vi "Top segment value_test3.vi"(10 "Top player segment position":string) -> (1 "Top player segment value":i32, 2 "Top player court segment display":bool[][](array[boolean]))   [LabVIEW 2014]
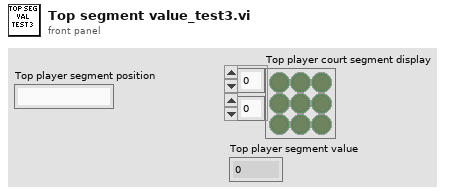
[diagram p1: front panel]
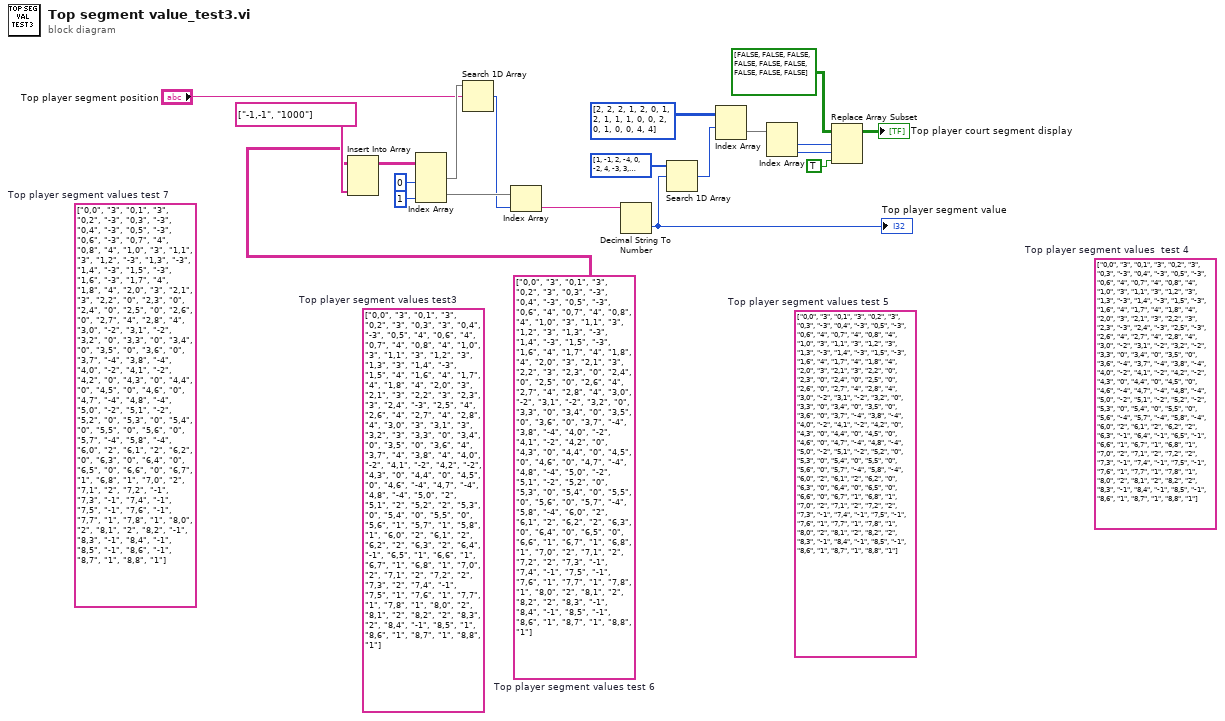
[diagram p0: block diagram]
diagram:
  (unwired) string[][] [["0,0", "3"], ["0,1", "3"], ["0,2", "-3"], ["0,3", "-3"], ["0,4", "-3"], ["0,5", "-3"], ["0,6", "-3"], ["0,7", "4"], ["0,8", "4"], ["1,0", "3"], ["1,1", "3"], ["1,2", "-3"], ["1,3", "-3"], ["1,4", "-3"], ["1,5", "-3"], ["1,6", "-3"], ["1,7", "4"], ["1,8", "4"], ["2,0", "3"], ["2,1", "3"], ["2,2", "0"], ["2,3", "0"], ["2,4", "0"], ["2,5", "0"], ["2,6", "0"], ["2,7", "4"], ["2,8", "4"], ["3,0", "-2"], ["3,1", "-2"], ["3,2", "0"], ["3,3", "0"], ["3,4", "0"], ["3,5", "0"], ["3,6", "0"], ["3,7", "-4"], ["3,8", "-4"], ["4,0", "-2"], ["4,1", "-2"], ["4,2", "0"], ["4,3", "0"], ["4,4", "0"], ["4,5", "0"], ["4,6", "0"], ["4,7", "-4"], ["4,8", "-4"], ["5,0", "-2"], ["5,1", "-2"], ["5,2", "0"], ["5,3", "0"], ["5,4", "0"], ["5,5", "0"], ["5,6", "0"], ["5,7", "-4"], ["5,8", "-4"], ["6,0", "2"], ["6,1", "2"], ["6,2", "0"], ["6,3", "0"], ["6,4", "0"], ["6,5", "0"], ["6,6", "0"], ["6,7", "1"], ["6,8", "1"], ["7,0", "2"], ["7,1", "2"], ["7,2", "-1"], ["7,3", "-1"], ["7,4", "-1"], ["7,5", "-1"], ["7,6", "-1"], ["7,7", "1"], ["7,8", "1"], ["8,0", "2"], ["8,1", "2"], ["8,2", "-1"], ["8,3", "-1"], ["8,4", "-1"], ["8,5", "-1"], ["8,6", "-1"], ["8,7", "1"], ["8,8", "1"]]  # Top player segment values test 7
  (unwired) string[][] [["0,0", "3"], ["0,1", "3"], ["0,2", "3"], ["0,3", "-3"], ["0,4", "-3"], ["0,5", "-3"], ["0,6", "4"], ["0,7", "4"], ["0,8", "4"], ["1,0", "3"], ["1,1", "3"], ["1,2", "3"], ["1,3", "-3"], ["1,4", "-3"], ["1,5", "-3"], ["1,6", "4"], ["1,7", "4"], ["1,8", "4"], ["2,0", "3"], ["2,1", "3"], ["2,2", "3"], ["2,3", "-3"], ["2,4", "-3"], ["2,5", "-3"], ["2,6", "4"], ["2,7", "4"], ["2,8", "4"], ["3,0", "-2"], ["3,1", "-2"], ["3,2", "-2"], ["3,3", "0"], ["3,4", "0"], ["3,5", "0"], ["3,6", "-4"], ["3,7", "-4"], ["3,8", "-4"], ["4,0", "-2"], ["4,1", "-2"], ["4,2", "-2"], ["4,3", "0"], ["4,4", "0"], ["4,5", "0"], ["4,6", "-4"], ["4,7", "-4"], ["4,8", "-4"], ["5,0", "-2"], ["5,1", "-2"], ["5,2", "-2"], ["5,3", "0"], ["5,4", "0"], ["5,5", "0"], ["5,6", "-4"], ["5,7", "-4"], ["5,8", "-4"], ["6,0", "2"], ["6,1", "2"], ["6,2", "2"], ["6,3", "-1"], ["6,4", "-1"], ["6,5", "-1"], ["6,6", "1"], ["6,7", "1"], ["6,8", "1"], ["7,0", "2"], ["7,1", "2"], ["7,2", "2"], ["7,3", "-1"], ["7,4", "-1"], ["7,5", "-1"], ["7,6", "1"], ["7,7", "1"], ["7,8", "1"], ["8,0", "2"], ["8,1", "2"], ["8,2", "2"], ["8,3", "-1"], ["8,4", "-1"], ["8,5", "-1"], ["8,6", "1"], ["8,7", "1"], ["8,8", "1"]]  # Top player segment values  test 4
  (unwired) string[][] [["0,0", "3"], ["0,1", "3"], ["0,2", "3"], ["0,3", "3"], ["0,4", "-3"], ["0,5", "4"], ["0,6", "4"], ["0,7", "4"], ["0,8", "4"], ["1,0", "3"], ["1,1", "3"], ["1,2", "3"], ["1,3", "3"], ["1,4", "-3"], ["1,5", "4"], ["1,6", "4"], ["1,7", "4"], ["1,8", "4"], ["2,0", "3"], ["2,1", "3"], ["2,2", "3"], ["2,3", "3"], ["2,4", "-3"], ["2,5", "4"], ["2,6", "4"], ["2,7", "4"], ["2,8", "4"], ["3,0", "3"], ["3,1", "3"], ["3,2", "3"], ["3,3", "0"], ["3,4", "0"], ["3,5", "0"], ["3,6", "4"], ["3,7", "4"], ["3,8", "4"], ["4,0", "-2"], ["4,1", "-2"], ["4,2", "-2"], ["4,3", "0"], ["4,4", "0"], ["4,5", "0"], ["4,6", "-4"], ["4,7", "-4"], ["4,8", "-4"], ["5,0", "2"], ["5,1", "2"], ["5,2", "2"], ["5,3", "0"], ["5,4", "0"], ["5,5", "0"], ["5,6", "1"], ["5,7", "1"], ["5,8", "1"], ["6,0", "2"], ["6,1", "2"], ["6,2", "2"], ["6,3", "2"], ["6,4", "-1"], ["6,5", "1"], ["6,6", "1"], ["6,7", "1"], ["6,8", "1"], ["7,0", "2"], ["7,1", "2"], ["7,2", "2"], ["7,3", "2"], ["7,4", "-1"], ["7,5", "1"], ["7,6", "1"], ["7,7", "1"], ["7,8", "1"], ["8,0", "2"], ["8,1", "2"], ["8,2", "2"], ["8,3", "2"], ["8,4", "-1"], ["8,5", "1"], ["8,6", "1"], ["8,7", "1"], ["8,8", "1"]]  # Top player segment values test3
  w2 = string[][] [["0,0", "3"], ["0,1", "3"], ["0,2", "3"], ["0,3", "-3"], ["0,4", "-3"], ["0,5", "-3"], ["0,6", "4"], ["0,7", "4"], ["0,8", "4"], ["1,0", "3"], ["1,1", "3"], ["1,2", "3"], ["1,3", "-3"], ["1,4", "-3"], ["1,5", "-3"], ["1,6", "4"], ["1,7", "4"], ["1,8", "4"], ["2,0", "3"], ["2,1", "3"], ["2,2", "3"], ["2,3", "0"], ["2,4", "0"], ["2,5", "0"], ["2,6", "4"], ["2,7", "4"], ["2,8", "4"], ["3,0", "-2"], ["3,1", "-2"], ["3,2", "0"], ["3,3", "0"], ["3,4", "0"], ["3,5", "0"], ["3,6", "0"], ["3,7", "-4"], ["3,8", "-4"], ["4,0", "-2"], ["4,1", "-2"], ["4,2", "0"], ["4,3", "0"], ["4,4", "0"], ["4,5", "0"], ["4,6", "0"], ["4,7", "-4"], ["4,8", "-4"], ["5,0", "-2"], ["5,1", "-2"], ["5,2", "0"], ["5,3", "0"], ["5,4", "0"], ["5,5", "0"], ["5,6", "0"], ["5,7", "-4"], ["5,8", "-4"], ["6,0", "2"], ["6,1", "2"], ["6,2", "2"], ["6,3", "0"], ["6,4", "0"], ["6,5", "0"], ["6,6", "1"], ["6,7", "1"], ["6,8", "1"], ["7,0", "2"], ["7,1", "2"], ["7,2", "2"], ["7,3", "-1"], ["7,4", "-1"], ["7,5", "-1"], ["7,6", "1"], ["7,7", "1"], ["7,8", "1"], ["8,0", "2"], ["8,1", "2"], ["8,2", "2"], ["8,3", "-1"], ["8,4", "-1"], ["8,5", "-1"], ["8,6", "1"], ["8,7", "1"], ["8,8", "1"]]  # Top player segment values test 6
  (unwired) string[][] [["0,0", "3"], ["0,1", "3"], ["0,2", "3"], ["0,3", "-3"], ["0,4", "-3"], ["0,5", "-3"], ["0,6", "4"], ["0,7", "4"], ["0,8", "4"], ["1,0", "3"], ["1,1", "3"], ["1,2", "3"], ["1,3", "-3"], ["1,4", "-3"], ["1,5", "-3"], ["1,6", "4"], ["1,7", "4"], ["1,8", "4"], ["2,0", "3"], ["2,1", "3"], ["2,2", "0"], ["2,3", "0"], ["2,4", "0"], ["2,5", "0"], ["2,6", "0"], ["2,7", "4"], ["2,8", "4"], ["3,0", "-2"], ["3,1", "-2"], ["3,2", "0"], ["3,3", "0"], ["3,4", "0"], ["3,5", "0"], ["3,6", "0"], ["3,7", "-4"], ["3,8", "-4"], ["4,0", "-2"], ["4,1", "-2"], ["4,2", "0"], ["4,3", "0"], ["4,4", "0"], ["4,5", "0"], ["4,6", "0"], ["4,7", "-4"], ["4,8", "-4"], ["5,0", "-2"], ["5,1", "-2"], ["5,2", "0"], ["5,3", "0"], ["5,4", "0"], ["5,5", "0"], ["5,6", "0"], ["5,7", "-4"], ["5,8", "-4"], ["6,0", "2"], ["6,1", "2"], ["6,2", "0"], ["6,3", "0"], ["6,4", "0"], ["6,5", "0"], ["6,6", "0"], ["6,7", "1"], ["6,8", "1"], ["7,0", "2"], ["7,1", "2"], ["7,2", "2"], ["7,3", "-1"], ["7,4", "-1"], ["7,5", "-1"], ["7,6", "1"], ["7,7", "1"], ["7,8", "1"], ["8,0", "2"], ["8,1", "2"], ["8,2", "2"], ["8,3", "-1"], ["8,4", "-1"], ["8,5", "-1"], ["8,6", "1"], ["8,7", "1"], ["8,8", "1"]]  # Top player segment values test 5
  n1 = Insert Into Array(array=w2, new element=string[] ["-1,-1", "1000"] ("new element/subarray")) -> (w13:string[][])  [unwired: 2 in]
  n2 = Index Array(array=w13, index (col) #1=0 ("disabled index (col)"), index (col) #2=1 ("index (col)")) -> (element #1=w19:string[], element #2=w16:string[])  [unwired: 2 in]
  n3 = Search 1D Array(1D array=w19, element="Top player segment position") -> (index of element=w15:i32)  [unwired: 1 in]
  n4 = Index Array(array=w16, index=w15) -> (element=w1:string)
  n5 = Decimal String To Number(string=w1) -> (number=w11:i32)  [unwired: 2 in, 1 out]
  "Top player segment value" <- w11
  n6 = Search 1D Array(1D array=i32[] [1, -1, 2, -4, 0, -2, 4, -3, 3, 1000], element=w11) -> (index of element=w9:i32)  [unwired: 1 in]
  n7 = Index Array(array=i32[][] [[2, 2], [2, 1], [2, 0], [1, 2], [1, 1], [1, 0], [0, 2], [0, 1], [0, 0], [4, 4]], index (row)=w9) -> (element=w8:i32[])  [unwired: 1 in]
  n8 = Index Array(array=w8) -> (element #1=w6:i32, element #2=w5:i32)  [unwired: 2 in]
  n9 = Replace Array Subset(array=bool[][] [[FALSE, FALSE, FALSE], [FALSE, FALSE, FALSE], [FALSE, FALSE, FALSE]] ("Top player court segment display"), new element=TRUE ("new element/subarray"), index (row)=w6, index (col)=w5) -> (→"Top player court segment display":bool[][])
